vi "HostHoppingScan_v2_IZTracked.vi"() -> ()   [LabVIEW 2024]
uses:
  <vilib>/Analysis/6fits.llb/Curve Fitting Criteria.ctl
  <vilib>/FPGAPlugInAG/USB-7845R OEM/niLvFpga_Open_USB-7845R OEM.vi
  <vilib>/rvi/interface/common/dynamic/niFpgaDynamicAddResources.vi
  <vilib>/Utility/error.llb/Error Cluster From Error Code.vi
  <vilib>/rvi/errors/niLvFpgaAdjustHostInterfaceError.vi
  <vilib>/FPGAPlugInAG/Dynamic/niLvFpga_Close_Dynamic.vi
  <vilib>/rvi/interface/common/niFpgaWaitOnOcc.vi
  <vilib>/rvi/interface/nirviOpenFPGA/nirviOpenFPGA.xnode
  FPGA Bitfiles/hoppingsicmv2_FPGATarget_FPGAScanningPrev_WLYS+VaKxTE.lvbitx
  <vilib>/rvi/interface/nirviReadWriteControl/nirviReadWriteControl.xnode
  <vilib>/rvi/interface/nirviCloseFPGA/nirviCloseFPGA.xnode
  FPGA Bitfiles/hoppingsicmv2_FPGATarget_FPGAHoppingScan_NADRfbve61k.lvbitx
  <vilib>/rvi/interface/nirviMethod/nirviMethod.xnode
  NiFpgaLv.dll
  <vilib>/rvi/interface/Simulation/niFpgaSimulationCallBeginRW.vi
  <vilib>/rvi/errors/niLvFpgaMergeErrorWithErrorCode.vi
  <vilib>/FPGAPlugInAG/Dynamic/niLvFpga_ReadFifo_Dynamic.vi
  <vilib>/FPGAPlugInAG/Dynamic/niLvFpga_WriteFifo_Dynamic.vi
  <vilib>/Analysis/NI_AALPro.lvlib
  <vilib>/FPGAPlugInAG/Dynamic/niLvFpga_ConfigureFifo_Dynamic.vi
panel:
  in  "SubstrateReference?":bool
  out "Signal Size":i32
  in  "Halting Threshold %":dbl format="%#_13g"
  in  "ScanPreview?":bool
  out "Done?":bool
  out "HTT_Buffer_Write":u32
  out "Scanned Points":i32
  in  "stop":bool
  in  "Notes":string
  in  "Pressure kPa":dbl format="%#_13g"
  in  "GraphTab":T1(tab)
  out "Topography":dbl[][](graph)
  out "IZCurve":cluster{dbl[], dbl[]}(graph)
  out "Pressure Slope Map":dbl[][](graph)
  out "FPGA_Host_Buf_Depth":u32
  in  "NF_AppRate um/s":dbl format="%#_13g"
  in  "FF_AppRate um/s":dbl format="%#_13g"
  in  "RetRate um/s":dbl format="%#_13g"
  in  "Retract um":dbl format="%#_13g"
  in  "XOffset um":dbl format="%#_13g"
  in  "YOffset um":dbl format="%#_13g"
  in  "YStepSize um":dbl format="%#_13g"
  in  "XStepSize um":dbl format="%#_13g"
  in  "Recording Threshold %":dbl format="%#_13g"
  in  "YNum":i32
  in  "XNum":i32
  in  "FrameNum":u32
  # "Put this down! ^^^"
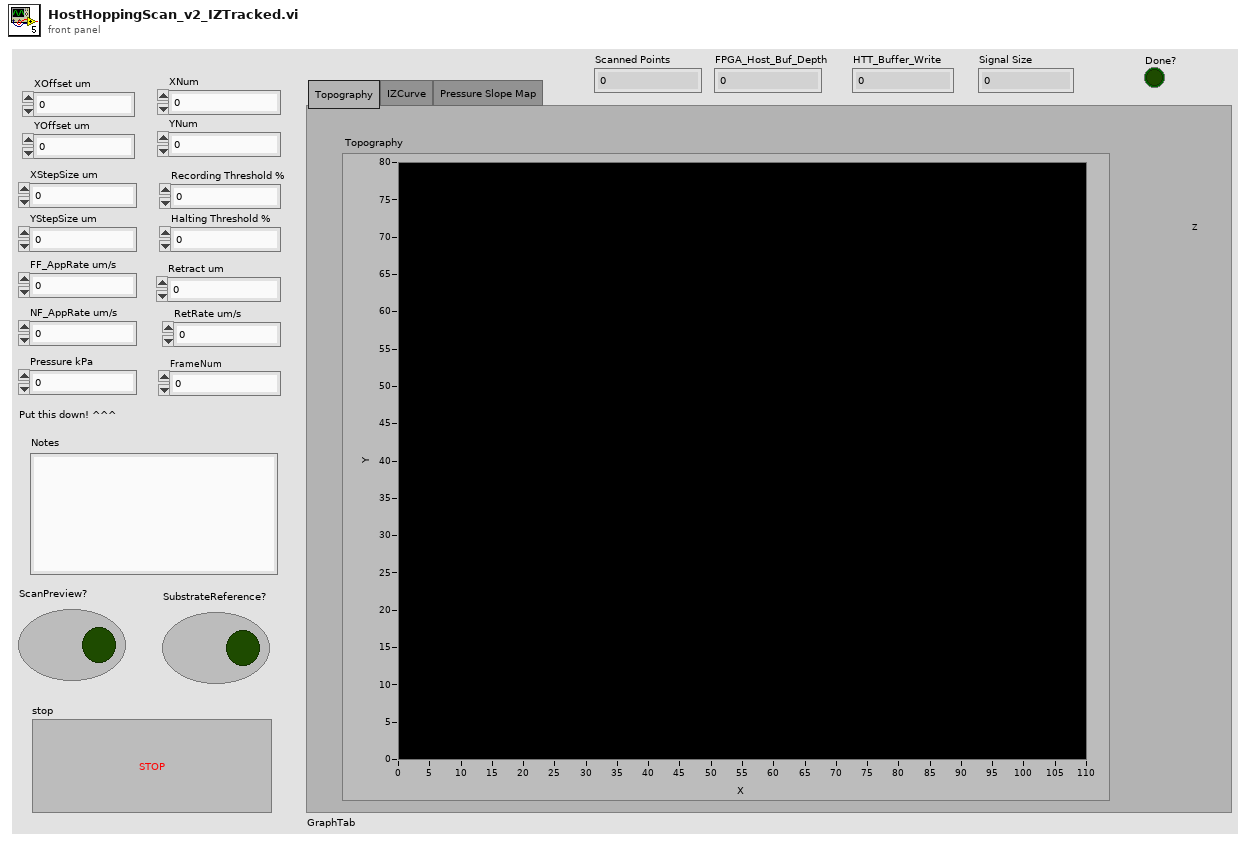
[diagram p1: front panel]
types:
  T1 = enum32{"Topography", "IZCurve", "Pressure Slope Map"}
  T2 = typedef "NI_AALPro.lvlib/Curve Fitting Criteria.ctl" = u16
diagram:
  n1 = flat-sequence {
    tunnel: [w4] -> w2
    tunnel: w2 -> [w14]
    tunnel: [w10] -> w1
    tunnel: w1 -> [w841]
    frame #0 {
      n2 = Obtain Queue(max queue size (-1, unlimited)=64, name (unnamed)="stop_sign", element data type=FALSE) -> (queue out=w4:refnum<queue>)  [unwired: 2 in, 2 out]
    }
    frame #1 {
      n3 = flat-sequence {
        tunnel: [w33] -> w15
        tunnel: w14 -> [w33]
        tunnel: w15 -> [w40]
        tunnel: [w40] -> w8
        tunnel: w8 -> [w104]
        tunnel: [w105] -> w7
        tunnel: [w114] -> w24
        tunnel: w7 -> [w113]
        tunnel: [w113] -> w13
        tunnel: w24 -> [w142]
        tunnel: [w124] -> w23
        tunnel: [w123] -> w22
        tunnel: [w121] -> w21
        tunnel: [w120] -> w20
        tunnel: w13 -> [w118]
        tunnel: [w118] -> w12
        tunnel: w23 -> [w155]
        tunnel: w22 -> [w154]
        tunnel: w21 -> [w153]
        tunnel: [w151] -> w19
        tunnel: [w150] -> w18
        tunnel: [w149] -> w17
        tunnel: [w148] -> w16
        tunnel: w20 -> [w152]
        tunnel: w12 -> [w147]
        tunnel: [w146] -> w11
        tunnel: w19 -> [w821]
        tunnel: w18 -> [w833]
        tunnel: w17 -> [w832]
        tunnel: w16 -> [w831]
        tunnel: w11 -> [w819]
        tunnel: [w819] -> w9
        tunnel: [w840] -> w10
        tunnel: w9 -> [w840]
        frame #0 {
          n4 = Wait (ms)(milliseconds to wait=u32 100) -> ()  [unwired: 1 out]
          "Done?" <- FALSE ("Done?")
        }
        frame #1 {
          n5 = local read "ScanPreview?"() -> (w35:bool)
          n6 = Get Queue Status(queue=w40) -> (queue out=w36:refnum<queue>, # elements in queue=w39:i32)  [unwired: 2 in, 6 out]
          n7 = Less Or Equal To 0?(x=w39) -> (x <= 0?=w38:bool)
          n8 = And(x=w35, y=w38) -> (x .and. y?=w37:bool)
          n9 = case shown="True" w37 {
            tunnel: w36 -> [_ w48]
            frame False {
            }
            frame True {
              n10 = flat-sequence {
                tunnel: w48 -> [w57]
                tunnel: [w56] -> w47
                tunnel: [w55] -> w46
                tunnel: [w57] -> w45
                tunnel: w47 -> [w83]
                tunnel: w46 -> [w82]
                tunnel: w45 -> [w84]
                tunnel: [w81] -> w44
                tunnel: [w80] -> w43
                tunnel: w44 -> [w97]
                tunnel: w43 -> [w96]
                tunnel: [w97] -> w42
                tunnel: [w96] -> w41
                tunnel: w42 -> [w100]
                tunnel: w41 -> [w99]
                frame #0 {
                  n11 = local read "YStepSize um"() -> (w61:dbl)
                  n12 = local read "XStepSize um"() -> (w69:dbl)
                  n13 = local read "YNum"() -> (w62:i32)
                  n14 = local read "XNum"() -> (w68:i32)
                  n15 = local read "XOffset um"() -> (w65:dbl)
                  n16 = local read "YOffset um"() -> (w60:dbl)
                  n17 = xnode "Open FPGA VI Reference"("resource name"=tag "RIO0") -> ("FPGA VI Reference Out"=w78:refnum<k20>, "error out"=w77:errorcluster)  [unwired: 1 in]
                  n18 = Decrement(x=w62) -> (x-1=w63:i32)
                  n19 = Decrement(x=w68) -> (x-1=w67:i32)
                  n20 = Multiply(x=w63, y=w61) -> (x*y=w64:dbl)
                  n21 = Multiply(x=w67, y=w69) -> (x*y=w66:dbl)
                  n22 = Add(x=w60, y=w64) -> (x+y=w50:dbl)
                  n23 = Add(x=w65, y=w66) -> (x+y=w53:dbl)
                  n24 = Divide(x=w50, y=10.0) -> (x/y=w49:dbl)
                  n25 = Divide(x=w53, y=10.0) -> (x/y=w52:dbl)
                  n26 = Divide(x=w60, y=10.0) -> (x/y=w72:dbl)
                  n27 = Divide(x=w65, y=10.0) -> (x/y=w74:dbl)
                  n28 = To Fixed-Point(number=w72) -> (fixed-point=w71:fxp<+/-,48,16>)  [unwired: 1 in]
                  n29 = To Fixed-Point(number=w49) -> (fixed-point=w58:fxp<+/-,48,16>)  [unwired: 1 in]
                  n30 = To Fixed-Point(number=w74) -> (fixed-point=w73:fxp<+/-,48,16>)  [unwired: 1 in]
                  n31 = To Fixed-Point(number=w52) -> (fixed-point=w59:fxp<+/-,48,16>)  [unwired: 1 in]
                  n32 = xnode "Read/Write Control"("FPGA VI Reference In"=w78, "error in"=w77, "X_start"=w73, "X_end"=w59, "Y_start"=w71, "Y_end"=w58, "rate us"=75) -> ("FPGA VI Reference Out"=w56:refnum<k20>, "error out"=w55:errorcluster)
                }
                frame #1 {
                  n33 = while {
                    tunnel: w84 -> [w95]
                    tunnel: w83 -> [w93]
                    tunnel: w82 -> [w92]
                    tunnel: [w91] -> w81
                    tunnel: [w90] -> w80
                    stop <- w85 stop-if-true
                    n34 = local read "ScanPreview?"() -> (w89:bool)
                    n35 = Get Queue Status(queue=w95) -> (# elements in queue=w94:i32)  [unwired: 2 in, 7 out]
                    n36 = Greater Than 0?(x=w94) -> (x > 0?=w88:bool)
                    n37 = Compound Arithmetic op=OR(invert w89, w88) -> (w87:bool)
                    n38 = xnode "Read/Write Control"("FPGA VI Reference In"=w93, "error in"=w92, "stop"=w87) -> ("FPGA VI Reference Out"=w91:refnum<k20>, "error out"=w90:errorcluster, "TargetDone?"=w85:bool)
                    n39 = Wait (ms)(milliseconds to wait=u32 10) -> ()  [unwired: 1 out]
                  }
                }
                frame #2 {
                  n40 = Wait (ms)(milliseconds to wait=u32 100) -> ()  [unwired: 1 out]
                }
                frame #3 {
                  n41 = xnode "Close FPGA VI Reference"("FPGA VI Reference In"=w100, "error in"=w99) -> ()  [unwired: 1 out]
                }
              }
            }
          }
        }
        frame #2 {
          n42 = Get Queue Status(queue=w104) -> (queue out=w103:refnum<queue>, # elements in queue=w102:i32)  [unwired: 2 in, 6 out]
          n43 = Greater Than 0?(x=w102) -> (x > 0?=w101:bool)
          n44 = case shown="True" w101 {
            tunnel: w103 -> [w107 w110]
            tunnel: [w107 w108] -> w105
            frame False {
            }
            frame True {
              n45 = flat-sequence {
                tunnel: w110 -> [w111]
                tunnel: [w111] -> w109
                tunnel: w109 -> [w112]
                tunnel: [w112] -> w108
                frame #0 {
                  n46 = Release Queue(queue=w111) -> ()  [unwired: 2 in, 3 out]
                }
                frame #1 {
                  n47 = Stop() -> ()  [unwired: 1 in]
                }
              }
            }
          }
          n48 = Wait (ms)(milliseconds to wait=u32 200) -> ()  [unwired: 1 out]
        }
        frame #3 {
          n49 = call "File Dialog"("prompt"="Choose a path to save scanning image data files") -> ("selected path"=w114:path, "cancelled"=w116:bool, "error out"=w115:errorcluster)  [unwired: 11 in, 1 out]
          n50 = Stop(stop? (T)=w116) -> ()
          n51 = call <vilib>:"Clear Errors.vi"("error in (no error)"=w115) -> ()  [unwired: 5 in, 2 out]
        }
        frame #4 {
          w127 = refnum<k38> refnum  # db_object
          # "use python to save data this time"
          n52 = Path To String(path=w142) -> (string=w141:string)
          n53 = Concatenate Strings(w141, "_data.db" ("string")) -> (w140:string)
          n54 = String To Path(string=w140) -> (path=w138:path)
          n55 = call <vilib>:"Check if File or Folder Exists.vi"("path"=w138) -> ("file or folder exists?"=w139:bool)  [unwired: 8 in, 2 out]
          n56 = Current VI's Path() -> (path=w132:path)
          n57 = case shown="True" w139 {
            tunnel: w138 -> [w143 w145]
            tunnel: [w143 w144] -> w137
            frame False {
            }
            frame True {
              n58 = Delete(path (use dialog)=w145) -> (deleted path=w144:path)  [unwired: 4 in, 2 out]
            }
          }
          n59 = Strip Path(path=w132) -> (stripped path=w131:path)  [unwired: 1 out]
          n60 = Path To String(path=w137) -> (string=w128:string)
          n61 = Build Path(base path=w131, name or relative path=path "py/data_db_arrangement.py") -> (appended path=w120:path)
          n62 = Open Python Session(python version="3.9" ("Python version")) -> (session out=w134:refnum<k35>, error out=w133:errorcluster)  [unwired: 2 in]
          n63 = node(w134, w120, "db_init" ("Python version"), w133, w127, w128) -> (w126:refnum<k35>, w125:errorcluster, w122:refnum<k38>)  [unwired: 1 in, 2 out]
          n64 = node(w126, w120, "db_start_global_timer" ("function name"), w125, w122) -> (w124:refnum<k35>, w123:errorcluster, w121:refnum<k38>)  [unwired: 2 in, 2 out]
        }
        frame #5 {
          n65 = local read "FrameNum"() -> (w156:u32)
          n66 = for {
            N: w156 -> [_]
            tunnel: w155 -> [w183]
            tunnel: w154 -> [w182]
            tunnel: w153 -> [w181]
            tunnel: w152 -> [w180]
            tunnel: [w169] -> w151
            tunnel: [w168] -> w150
            tunnel: [w167] -> w149
            tunnel: [w166] -> w148
            tunnel: w147 -> [w162]
            tunnel: [w159] -> w146
            i -> [w179]
            stop <- w163 stop-if-true
            n67 = flat-sequence {
              tunnel: w179 -> [w197]
              tunnel: w180 -> [w190]
              tunnel: w181 -> [w192]
              tunnel: w182 -> [w193]
              tunnel: w183 -> [w194]
              tunnel: [w191] -> w178
              tunnel: [w189] -> w177
              tunnel: [w188] -> w176
              tunnel: [w190] -> w175
              tunnel: [w197] -> w174
              tunnel: w162 -> [w186]
              tunnel: [w186] -> w161
              tunnel: [w237] -> w184
              tunnel: w178 -> [w232]
              tunnel: w177 -> [w231]
              tunnel: w176 -> [w230]
              tunnel: w175 -> [w229]
              tunnel: w174 -> [w228]
              tunnel: [w223] -> w173
              tunnel: [w222] -> w172
              tunnel: [w221] -> w171
              tunnel: [w220] -> w170
              tunnel: [w219] -> w165
              tunnel: [w218] -> w164
              tunnel: w161 -> [w208]
              tunnel: [w207] -> w160
              tunnel: [w203] -> w158
              tunnel: [w202] -> w157
              tunnel: w184 -> [w810]
              tunnel: w173 -> [w805]
              tunnel: w172 -> [w807]
              tunnel: w171 -> [w806]
              tunnel: w170 -> [w802]
              tunnel: [w805] -> w169
              tunnel: [w804] -> w168
              tunnel: [w803] -> w167
              tunnel: [w801] -> w166
              tunnel: w165 -> [w808]
              tunnel: w164 -> [w809]
              tunnel: [w809] -> w163
              tunnel: w160 -> [w799]
              tunnel: [w799] -> w159
              tunnel: w158 -> [w797]
              tunnel: w157 -> [w798]
              frame #0 {
                w185 = FALSE ("Y Scale.Loose Fit")
                n68 = local read "XNum"() -> (w196:i32)
                n69 = local read "YNum"() -> (w195:i32)
                n70 = property on="Pressure Slope Map" class="IntGraph (strict)"("XScale.Maximum"=w196, "YScale.Maximum"=w195, "YScale.LooseFit"=w185, "XScale.LooseFit"=w185, "ZScale.LooseFit"=w185) -> ()  [unwired: 2 in, 2 out]
                n71 = property on="Topography" class="IntGraph (strict)"("XScale.Maximum"=w196, "YScale.Maximum"=w195, "YScale.LooseFit"=w185, "XScale.LooseFit"=w185, "ZScale.LooseFit"=w185) -> ()  [unwired: 2 in, 2 out]
                n72 = node(w194, w190, "db_start_frame_timer" ("function name"), w193, w192) -> (w191:refnum<k35>, w189:errorcluster, w188:refnum<k38>)  [unwired: 2 in, 2 out]
              }
              frame #1 {
                w200 = 100000.0
                w201 = -100000.0
                # "TTH param structure:\n0, 1: X, Y piezo voltage\n2, 3: X, Y piezo idx\n4: Z piezo voltage\n5: baseline current\n(6-8105): Z voltage\n(8106-16205): current"
                # "HTT param structure:\n0, 1: X, Y piezo voltage\n2, 3: X, Y piezo idx\n4: distance (piezo voltage) to the last point\n5: retract height, \nall negative cases won't trigger approach of z piezo\nif -20, keep z and move xy\nif -30, full retract for z and move xy"
                n73 = Obtain Queue(name (unnamed)="data_array", element data type=dbl[] []) -> (queue out=w233:refnum<queue>)  [unwired: 3 in, 2 out]
                n74 = New Data Value Reference(data value=FALSE) -> (data value reference=w234:refnum<data-value>)  [unwired: 1 in, 1 out]
                n75 = local read "XNum"() -> (w226:i32)
                n76 = local read "YNum"() -> (w225:i32)
                n77 = Initialize Array(0.0, w226, w225) -> (w224:dbl[][])
                n78 = flat-sequence {
                  tunnel: w234 -> [w560]
                  tunnel: w233 -> [w561]
                  tunnel: [w561] -> w258
                  tunnel: [w560] -> w256
                  tunnel: [w559] -> w254
                  tunnel: [w551] -> w251
                  tunnel: [w545] -> w245
                  tunnel: [w542] -> w244
                  tunnel: [w536] -> w243
                  tunnel: [w533] -> w242
                  tunnel: [w532] -> w199
                  tunnel: [w522] -> w198
                  tunnel: [w583] -> w260
                  tunnel: [w582] -> w259
                  tunnel: w258 -> [w581]
                  tunnel: [w581] -> w257
                  tunnel: w256 -> [w574]
                  tunnel: [w574] -> w255
                  tunnel: w254 -> [w564]
                  tunnel: [w576] -> w253
                  tunnel: [w575] -> w252
                  tunnel: w251 -> [w573]
                  tunnel: [w573] -> w250
                  tunnel: [w574] -> w249
                  tunnel: [w572] -> w248
                  tunnel: [0] -> w247
                  tunnel: [w570] -> w246
                  tunnel: w245 -> [w569]
                  tunnel: w244 -> [w568]
                  tunnel: w243 -> [w567]
                  tunnel: w242 -> [w565]
                  tunnel: [0] -> w236
                  tunnel: [w565] -> w235
                  tunnel: w199 -> [w563]
                  tunnel: w198 -> [w562]
                  tunnel: w260 -> [w609]
                  tunnel: w259 -> [w608]
                  tunnel: w257 -> [w607]
                  tunnel: w255 -> [w606]
                  tunnel: w253 -> [w605]
                  tunnel: w252 -> [w604]
                  tunnel: w250 -> [w603]
                  tunnel: w249 -> [w602]
                  tunnel: w248 -> [w601]
                  tunnel: w247 -> [w600]
                  tunnel: w246 -> [w599]
                  tunnel: [w598] -> w241
                  tunnel: [w597] -> w240
                  tunnel: [w596] -> w239
                  tunnel: [w595] -> w238
                  tunnel: w236 -> [w594]
                  tunnel: w235 -> [w593]
                  tunnel: [w592] -> w217
                  tunnel: [w591] -> w206
                  tunnel: [w775] -> w216
                  tunnel: [w774] -> w214
                  tunnel: [w773] -> w212
                  tunnel: [w771] -> w210
                  tunnel: w217 -> [w770]
                  tunnel: w238 -> [w772]
                  tunnel: w239 -> [w773]
                  tunnel: w240 -> [w774]
                  tunnel: w241 -> [w775]
                  tunnel: w206 -> [w769]
                  tunnel: [w769] -> w204
                  tunnel: w216 -> [w789]
                  tunnel: [w789] -> w215
                  tunnel: w214 -> [w788]
                  tunnel: [w788] -> w213
                  tunnel: w212 -> [w787]
                  tunnel: [w787] -> w211
                  tunnel: w210 -> [w786]
                  tunnel: [w786] -> w209
                  tunnel: [w784] -> w205
                  tunnel: w204 -> [w784]
                  tunnel: w215 -> [w794]
                  tunnel: w213 -> [w793]
                  tunnel: w211 -> [w795]
                  tunnel: w209 -> [w792]
                  tunnel: [w792] -> w237
                  tunnel: [w791] -> w219
                  tunnel: w205 -> [w790]
                  tunnel: [w790] -> w203
                  frame #0 {
                    n79 = local read "NF_AppRate um/s"() -> (w543:dbl)
                    n80 = local read "FF_AppRate um/s"() -> (w548:dbl)
                    n81 = local read "Recording Threshold %"() -> (w531:dbl)
                    n82 = local read "SubstrateReference?"() -> (w525:bool)
                    n83 = local read "Halting Threshold %"() -> (w527:dbl)
                    n84 = local read "RetRate um/s"() -> (w538:dbl)
                    n85 = local read "XNum"() -> (w535:i32)
                    n86 = local read "YNum"() -> (w534:i32)
                    n87 = Divide(x=25.0, y=0.032768) -> (x/y=w537:dbl)
                    n88 = local read "XStepSize um"() -> (w556:dbl)
                    n89 = local read "YStepSize um"() -> (w555:dbl)
                    n90 = local read "YOffset um"() -> (w554:dbl)
                    n91 = local read "Retract um"() -> (w552:dbl)
                    n92 = local read "XOffset um"() -> (w553:dbl)
                    n93 = local read "XNum"() -> (w558:i32)
                    n94 = local read "YNum"() -> (w557:i32)
                    n95 = Multiply(x=w535, y=w534) -> (x*y=w533:i32)
                    n96 = Divide(x=w531, y=100.0) -> (x/y=w530:dbl)
                    n97 = Divide(x=w527, y=100.0) -> (x/y=w526:dbl)
                    n98 = Divide(x=w537, y=w543) -> (x/y=w539:dbl)
                    n99 = Divide(x=w537, y=w538) -> (x/y=w541:dbl)
                    n100 = Divide(x=w537, y=w548) -> (x/y=w547:dbl)
                    n101 = Round To Nearest(number=w539) -> (nearest integer value=w544:dbl)
                    n102 = Round To Nearest(number=w541) -> (nearest integer value=w540:dbl)
                    n103 = Round To Nearest(number=w547) -> (nearest integer value=w546:dbl)
                    n104 = To Fixed-Point(number=w530) -> (fixed-point=w559:fxp<+/-,48,16>)  [unwired: 1 in]
                    n105 = To Fixed-Point(number=w526) -> (fixed-point=w532:fxp<+/-,48,16>)  [unwired: 1 in]
                    n106 = call "xy_raster_scan.vi"("Retract um"=w552, "YOffset um"=w554, "XOffset um"=w553, "YStepSize um"=w555, "XStepSize um"=w556, "YNum"=w557, "XNum"=w558) -> ("Converted_HTT_Params"=w551:fxp<+/-,48,16>[])  [unwired: 4 in]
                    n107 = Select(t=2, s=w525, f=1) -> (s? t:f=w522:i32)
                    n108 = To Long Integer(number=w544) -> (32bit integer=w542:i32)
                    n109 = To Long Integer(number=w540) -> (32bit integer=w536:i32)
                    n110 = To Long Integer(number=w546) -> (32bit integer=w545:i32)
                  }
                  frame #1 {
                    n111 = xnode "Open FPGA VI Reference"("resource name"=tag "RIO0") -> ("FPGA VI Reference Out"=w580:refnum<k20>, "error out"=w579:errorcluster)  [unwired: 1 in]
                    n112 = xnode "Read/Write Control"("FPGA VI Reference In"=w580, "error in"=w579, "Recording Threshold"=w564, "Halting Threshold"=w563, "AppRate_FF us"=w569, "AppRate_NF us"=w568, "RetRate us"=w567, "TotalPoints"=w565, "DelayPoints"=w562) -> ("FPGA VI Reference Out"=w589:refnum<k20>, "error out"=w588:errorcluster)
                    n113 = xnode "Invoke Method"("FPGA VI Reference In"=w580, "error in"=w579, "Data"=fxp<+/-,48,16>[] [], "Timeout (ms)"=0) -> ("FPGA VI Reference Out"=w576:refnum<k20>, "error out"=w575:errorcluster, "Empty Elements Remaining"=w570:u32)
                    n114 = Scale By Power Of 2(n=u32 18 ("Requested Depth"), x=u32 1 ("Requested Depth")) -> (x*2^n=w585:u32)
                    n115 = xnode "Invoke Method"("FPGA VI Reference In"=w589, "error in"=w588, "Requested Depth"=w585) -> ("FPGA VI Reference Out"=w583:refnum<k20>, "error out"=w582:errorcluster, "Actual Depth"=→"FPGA_Host_Buf_Depth":u32)
                    n116 = Array Size(array=w573) -> (size(s)=w572:i32)
                  }
                  frame #2 {
                    n117 = while {
                      tunnel: w605 -> [w627]
                      tunnel: w604 -> [w626]
                      tunnel: w603 -> [w623]
                      tunnel: w602 -> [w622]
                      tunnel: w601 -> [w621]
                      shift-right: [w614] -> _
                      shift-left: w600 -> [w620]
                      tunnel: w599 -> [w619]
                      stop <- w610 stop-if-true
                      n118 = flat-sequence {
                        tunnel: w627 -> [w651]
                        tunnel: w626 -> [w650]
                        tunnel: [w645] -> w625
                        tunnel: [w644] -> w624
                        tunnel: w623 -> [w633]
                        tunnel: w622 -> [w643]
                        tunnel: w621 -> [w642]
                        tunnel: w620 -> [w637]
                        tunnel: w619 -> [w641]
                        tunnel: [w637] -> w618
                        tunnel: [w634] -> w617
                        tunnel: [w633] -> w616
                        tunnel: [w629] -> w613
                        tunnel: [w628] -> w612
                        tunnel: w625 -> [w660]
                        tunnel: w624 -> [w659]
                        tunnel: w618 -> [w658]
                        tunnel: w617 -> [w657]
                        tunnel: w616 -> [w656]
                        tunnel: [w655] -> w615
                        tunnel: w613 -> [w654]
                        tunnel: w612 -> [w653]
                        tunnel: [w653] -> w611
                        tunnel: w615 -> [w671]
                        tunnel: [w671] -> w614
                        tunnel: w611 -> [w670]
                        tunnel: [w670] -> w610
                        frame #0 {
                          w635 = u32 128 ("y")
                          n119 = in-place {
                            in-place-border: [w652] -> w631
                            n120 = in-place-dvr #1(w643) -> (w652:bool)  [unwired: 1 out]
                            n121 = in-place-dvr #1(w652) -> ()  [unwired: 2 out]
                          }
                          n122 = xnode "Invoke Method"("FPGA VI Reference In"=w651, "error in"=w650, "Data"=fxp<+/-,48,16>[] [], "Timeout (ms)"=0) -> ("FPGA VI Reference Out"=w647:refnum<k20>, "error out"=w646:errorcluster, "Empty Elements Remaining"=w640:u32)
                          n123 = Subtract(x=w642, y=w637) -> (x-y=w636:u32)
                          n124 = Subtract(x=w641, y=w640) -> (x-y=w639:u32)
                          n125 = Less Or Equal?(x=w639, y=w635) -> (x <= y?=w638:bool)
                          n126 = Less Or Equal?(x=w636, y=w635) -> (x <= y?=w630:bool)
                          n127 = Or(x=w638, y=w630) -> (x .or. y?=w629:bool)
                          n128 = xnode "Read/Write Control"("FPGA VI Reference In"=w647, "error in"=w646) -> ("FPGA VI Reference Out"=w645:refnum<k20>, "error out"=w644:errorcluster, "TargetDone?"=w632:bool)
                          n129 = Select(t=w636, s=w630, f=w635) -> (s? t:f=w634:u32)
                          n130 = Compound Arithmetic op=OR(w632, w630, w631) -> (w628:bool)
                        }
                        frame #1 {
                          n131 = case shown="True" w654 {
                            tunnel: w660 -> [_ w669]
                            tunnel: w659 -> [_ w668]
                            tunnel: w658 -> [w661 w664]
                            tunnel: w657 -> [_ w663]
                            tunnel: w656 -> [_ w665]
                            tunnel: [w661 w666] -> w655
                            frame False {
                            }
                            frame True {
                              n132 = Array Subset(array=w665, index=w664, length=w663) -> (w662:fxp<+/-,48,16>[])
                              n133 = Add(x=w663, y=w664) -> (x+y=w666:u32)
                              "HTT_Buffer_Write" <- w666
                              n134 = xnode "Invoke Method"("FPGA VI Reference In"=w669, "error in"=w668, "Data"=w662, "Timeout (ms)"=10000) -> ()  [unwired: 3 out]
                            }
                          }
                        }
                        frame #2 {
                          n135 = Wait (ms)(milliseconds to wait=u32 100) -> ()  [unwired: 1 out]
                        }
                      }
                    }
                    n136 = while {
                      tunnel: w609 -> [w702]
                      tunnel: w608 -> [w701]
                      tunnel: w607 -> [w698]
                      tunnel: w606 -> [w697]
                      tunnel: [w690] -> w598
                      tunnel: [w689] -> w597
                      tunnel: [w687] -> w596
                      tunnel: [w685] -> w595
                      shift-right: [w681] -> _
                      shift-left: w594 -> [w684]
                      tunnel: w593 -> [w677]
                      tunnel: [w674] -> w592
                      tunnel: [w673] -> w591
                      stop <- w678 stop-if-true
                      n137 = flat-sequence {
                        tunnel: w702 -> [w721]
                        tunnel: w701 -> [w720]
                        tunnel: [w715] -> w700
                        tunnel: [w714] -> w699
                        tunnel: w698 -> [w710]
                        tunnel: w697 -> [w708]
                        tunnel: [w710] -> w696
                        tunnel: [w709] -> w695
                        tunnel: [w707] -> w694
                        tunnel: [w706] -> w691
                        tunnel: w684 -> [w705]
                        tunnel: [w705] -> w683
                        tunnel: [w704] -> w680
                        tunnel: w677 -> [w703]
                        tunnel: [w703] -> w676
                        tunnel: w700 -> [w735]
                        tunnel: w699 -> [w734]
                        tunnel: w696 -> [w733]
                        tunnel: w695 -> [w732]
                        tunnel: w694 -> [w731]
                        tunnel: [w730] -> w693
                        tunnel: [w729] -> w692
                        tunnel: w691 -> [w728]
                        tunnel: [w728] -> w688
                        tunnel: [w727] -> w686
                        tunnel: w683 -> [w726]
                        tunnel: [w725] -> w682
                        tunnel: w680 -> [w724]
                        tunnel: [w724] -> w679
                        tunnel: w676 -> [w723]
                        tunnel: [w723] -> w675
                        tunnel: w693 -> [w767]
                        tunnel: w692 -> [w766]
                        tunnel: [w767] -> w690
                        tunnel: [w766] -> w689
                        tunnel: [w765] -> w687
                        tunnel: w688 -> [w765]
                        tunnel: w686 -> [w764]
                        tunnel: [w764] -> w685
                        tunnel: w682 -> [w762]
                        tunnel: [w762] -> w681
                        tunnel: w679 -> [w760]
                        tunnel: [w763] -> w678
                        tunnel: w675 -> [w761]
                        tunnel: [w760] -> w674
                        tunnel: [w759] -> w673
                        frame #0 {
                          w713 = 16384
                          w717 = u32 0 ("Number of Elements")
                          n138 = in-place {
                            in-place-border: [w722] -> w704
                            n139 = in-place-dvr #2(w708) -> (w722:bool)  [unwired: 1 out]
                            n140 = in-place-dvr #2(w722) -> (w706:refnum<data-value>)  [unwired: 1 out]
                          }
                          n141 = xnode "Read/Write Control"("FPGA VI Reference In"=w721, "error in"=w720, "stop"=w704) -> ("FPGA VI Reference Out"=w719:refnum<k20>, "error out"=w718:errorcluster)
                          n142 = xnode "Invoke Method"("FPGA VI Reference In"=w719, "error in"=w718, "Number of Elements"=w717, "Timeout (ms)"=w717) -> ("FPGA VI Reference Out"=w715:refnum<k20>, "error out"=w714:errorcluster, "Elements Remaining"=w716:u32)  [unwired: 1 out]
                          n143 = Quotient & Remainder(x=w716, y=w713) -> (floor(x/y)=w712:u32)  [unwired: 1 out]
                          n144 = Multiply(x=w713, y=w712) -> (x*y=w707:u32)
                          n145 = Greater Than 0?(x=w712) -> (x > 0?=w711:bool)
                          n146 = Compound Arithmetic op=AND(w711, invert w704) -> (w709:bool)
                        }
                        frame #1 {
                          n147 = case shown="True" w732 {
                            tunnel: w735 -> [w739 w755]
                            tunnel: w734 -> [w738 w754]
                            tunnel: w733 -> [w737 w748]
                            tunnel: w731 -> [_ w750]
                            tunnel: [w739 w752] -> w730
                            tunnel: [w738 w751] -> w729
                            tunnel: [w737 w743] -> w727
                            tunnel: w726 -> [w736 w742]
                            tunnel: [w736 w740] -> w725
                            frame False {
                            }
                            frame True {
                              w745 = 16384
                              n148 = xnode "Invoke Method"("FPGA VI Reference In"=w755, "error in"=w754, "Number of Elements"=w750, "Timeout (ms)"=10000) -> ("FPGA VI Reference Out"=w752:refnum<k20>, "error out"=w751:errorcluster, "Data"=w749:fxp<+/-,48,16>[])  [unwired: 1 out]
                              n149 = To Double Precision Float(number=w749) -> (double precision float=w746:dbl[])
                              n150 = Array Size(array=w746) -> (size(s)=w747:i32)
                              n151 = Quotient & Remainder(x=w747, y=w745) -> (floor(x/y)=w741:i32)  [unwired: 1 out]
                              n152 = Add(x=w742, y=w741) -> (x+y=w740:i32)
                              n153 = Reshape Array(w746, w741, w745) -> (w744:dbl[][])
                              n154 = for {
                                N: w741 -> [_]
                                tunnel: w748 -> [w758]
                                tunnel: w744 -> [w757] mode=indexing
                                tunnel: [w756] -> w743
                                n155 = Enqueue Element(queue=w758, element=w757) -> (queue out=w756:refnum<queue>)  [unwired: 2 in, 2 out]
                              }
                            }
                          }
                        }
                        frame #2 {
                          n156 = Greater Or Equal?(x=w762, y=w761) -> (x >= y?=w759:bool)
                          n157 = Wait (ms)(milliseconds to wait=u32 20) -> ()  [unwired: 1 out]
                          n158 = Or(x=w759, y=w760) -> (x .or. y?=w763:bool)
                          "Scanned Points" <- w762
                        }
                      }
                    }
                  }
                  frame #3 {
                    n159 = case shown="False" w770 {
                      tunnel: w772 -> [w777 w783]
                      tunnel: [w776 w783] -> w771
                      frame False {
                        n160 = while {
                          tunnel: w777 -> [w782]
                          tunnel: [w781] -> w776
                          stop <- w779 stop-if-true
                          n161 = Get Queue Status(queue=w782) -> (queue out=w781:refnum<queue>, # elements in queue=w780:i32)  [unwired: 2 in, 6 out]
                          n162 = Less Or Equal To 0?(x=w780) -> (x <= 0?=w779:bool)
                          n163 = Wait (ms)(milliseconds to wait=u32 100) -> ()  [unwired: 1 out]
                        }
                      }
                      frame True {
                      }
                    }
                  }
                  frame #4 {
                    n164 = Wait (ms)(milliseconds to wait=u32 500) -> ()  [unwired: 1 out]
                  }
                  frame #5 {
                    n165 = in-place {
                      n166 = in-place-dvr #3(w795) -> ()  [unwired: 2 out]
                      n167 = in-place-dvr #3(TRUE ("data value")) -> (w791:refnum<data-value>)  [unwired: 1 out]
                    }
                    n168 = xnode "Close FPGA VI Reference"("FPGA VI Reference In"=w794, "error in"=w793) -> ()  [unwired: 1 out]
                  }
                }
                n169 = flat-sequence {
                  tunnel: w234 -> [w284]
                  tunnel: w233 -> [w283]
                  tunnel: w232 -> [w282]
                  tunnel: w231 -> [w281]
                  tunnel: w230 -> [w280]
                  tunnel: w229 -> [w279]
                  tunnel: [w278] -> w223
                  tunnel: [w277] -> w222
                  tunnel: [w276] -> w221
                  tunnel: [w275] -> w220
                  tunnel: w228 -> [w274]
                  tunnel: w224 -> [w273]
                  tunnel: w224 -> [w272]
                  tunnel: w201 -> [w271]
                  tunnel: w200 -> [w270]
                  tunnel: w201 -> [w269]
                  tunnel: w200 -> [w268]
                  tunnel: [w267] -> w218
                  tunnel: w208 -> [w266]
                  tunnel: [w265] -> w207
                  tunnel: [w264] -> w202
                  frame #0 {
                    n170 = while {
                      tunnel: w284 -> [w343]
                      tunnel: w283 -> [w342]
                      tunnel: w282 -> [w341]
                      tunnel: w281 -> [w340]
                      tunnel: w280 -> [w339]
                      tunnel: w279 -> [w335]
                      tunnel: [w329] -> w278
                      tunnel: [w328] -> w277
                      tunnel: [w327] -> w276
                      tunnel: [w326] -> w275
                      tunnel: w274 -> [w322]
                      shift-right: [w312] -> _
                      shift-left: w273 -> [w320]
                      shift-right: [w310] -> _
                      shift-left: w272 -> [w315]
                      shift-right: [w300] -> _
                      shift-left: w271 -> [w309]
                      shift-right: [w298] -> _
                      shift-left: w270 -> [w308]
                      shift-right: [w296] -> _
                      shift-left: w269 -> [w305]
                      shift-right: [w294] -> _
                      shift-left: w268 -> [w304]
                      tunnel: [w291] -> w267
                      tunnel: w266 -> [w290]
                      tunnel: [w287] -> w265
                      tunnel: [w285] -> w264
                      stop <- w317 stop-if-true
                      n171 = flat-sequence {
                        tunnel: w343 -> [w365]
                        tunnel: w342 -> [w360]
                        tunnel: w341 -> [w364]
                        tunnel: w340 -> [w363]
                        tunnel: w339 -> [w362]
                        tunnel: [w364] -> w338
                        tunnel: [w363] -> w337
                        tunnel: [w362] -> w336
                        tunnel: w335 -> [w361]
                        tunnel: [w361] -> w334
                        tunnel: [w359] -> w325
                        tunnel: [w358] -> w324
                        tunnel: [w357] -> w323
                        tunnel: w322 -> [w356]
                        tunnel: [w356] -> w321
                        tunnel: w320 -> [w354]
                        tunnel: [w355] -> w319
                        tunnel: [w354] -> w316
                        tunnel: w315 -> [w353]
                        tunnel: [w353] -> w314
                        tunnel: w309 -> [w352]
                        tunnel: w308 -> [w351]
                        tunnel: [w352] -> w307
                        tunnel: [w351] -> w306
                        tunnel: w305 -> [w350]
                        tunnel: w304 -> [w349]
                        tunnel: [w350] -> w303
                        tunnel: [w349] -> w302
                        tunnel: [w348] -> w293
                        tunnel: w290 -> [w347]
                        tunnel: [w344] -> w289
                        tunnel: w338 -> [w396]
                        tunnel: w337 -> [w395]
                        tunnel: w336 -> [w394]
                        tunnel: w334 -> [w393]
                        tunnel: [w392] -> w333
                        tunnel: [w391] -> w332
                        tunnel: [w390] -> w331
                        tunnel: [w389] -> w330
                        tunnel: w325 -> [w388]
                        tunnel: w324 -> [w387]
                        tunnel: w323 -> [w386]
                        tunnel: w321 -> [w385]
                        tunnel: w319 -> [w384]
                        tunnel: [w384] -> w318
                        tunnel: w316 -> [w383]
                        tunnel: w314 -> [w382]
                        tunnel: [w381] -> w313
                        tunnel: [w380] -> w311
                        tunnel: w307 -> [w379]
                        tunnel: w306 -> [w378]
                        tunnel: w303 -> [w377]
                        tunnel: w302 -> [w376]
                        tunnel: [w375] -> w301
                        tunnel: [w374] -> w299
                        tunnel: [w373] -> w297
                        tunnel: [w372] -> w295
                        tunnel: w293 -> [w371]
                        tunnel: [w371] -> w292
                        tunnel: w289 -> [w370]
                        tunnel: [w370] -> w288
                        tunnel: [w369] -> w286
                        tunnel: w333 -> [w519]
                        tunnel: w332 -> [w518]
                        tunnel: w331 -> [w517]
                        tunnel: w330 -> [w520]
                        tunnel: [w520] -> w329
                        tunnel: [w519] -> w328
                        tunnel: [w518] -> w327
                        tunnel: [w517] -> w326
                        tunnel: [w516] -> w317
                        tunnel: w318 -> [w516]
                        tunnel: w313 -> [w515]
                        tunnel: [w515] -> w312
                        tunnel: w311 -> [w514]
                        tunnel: [w514] -> w310
                        tunnel: w301 -> [w513]
                        tunnel: [w513] -> w300
                        tunnel: w299 -> [w512]
                        tunnel: [w512] -> w298
                        tunnel: w297 -> [w511]
                        tunnel: [w511] -> w296
                        tunnel: w295 -> [w510]
                        tunnel: [w510] -> w294
                        tunnel: w292 -> [w509]
                        tunnel: [w509] -> w291
                        tunnel: w288 -> [w508]
                        tunnel: [w508] -> w287
                        tunnel: w286 -> [w507]
                        tunnel: [w507] -> w285
                        frame #0 {
                          # "topography max min"
                          # "pressure slope map"
                          # "topography"
                          n172 = Get Queue Status(queue=w347) -> (queue out=w344:refnum<queue>, # elements in queue=w346:i32)  [unwired: 2 in, 6 out]
                          n173 = Greater Than 0?(x=w346) -> (x > 0?=w345:bool)
                          n174 = Get Queue Status(queue=w360) -> (queue out=w358:refnum<queue>, # elements in queue=w357:i32)  [unwired: 2 in, 6 out]
                          n175 = in-place {
                            in-place-border: w345 -> [w366]
                            in-place-border: [w367] -> w355
                            in-place-border: [w366] -> w348
                            n176 = in-place-dvr #4(w365) -> (w368:bool)  [unwired: 1 out]
                            n177 = Or(x=w368, y=w366) -> (x .or. y?=w367:bool)
                            n178 = in-place-dvr #4(w367) -> ()  [unwired: 2 out]
                          }
                          n179 = Greater Than 0?(x=w357) -> (x > 0?=w359:bool)
                        }
                        frame #1 {
                          n180 = case shown="True" w388 {
                            tunnel: w396 -> [w406 w434]
                            tunnel: w395 -> [w405 w433]
                            tunnel: w394 -> [w404 w432]
                            tunnel: w393 -> [w407 w428]
                            tunnel: [w406 w431] -> w392
                            tunnel: [w405 w430] -> w391
                            tunnel: [w404 w429] -> w390
                            tunnel: [w407 w427] -> w389
                            tunnel: w387 -> [_ w425]
                            tunnel: w386 -> [_ w426]
                            tunnel: w385 -> [w397 w424]
                            tunnel: w383 -> [w403 w423]
                            tunnel: w382 -> [w402 w422]
                            tunnel: [w403 w421] -> w381
                            tunnel: [w402 w420] -> w380
                            tunnel: w379 -> [w401 w416]
                            tunnel: w378 -> [w400 w415]
                            tunnel: w377 -> [w399 w414]
                            tunnel: w376 -> [w398 w413]
                            tunnel: [w401 w412] -> w375
                            tunnel: [w400 w411] -> w374
                            tunnel: [w399 w410] -> w373
                            tunnel: [w398 w409] -> w372
                            tunnel: [w397 w408] -> w369
                            frame False {
                            }
                            frame True {
                              n181 = for {
                                N: w426 -> [_]
                                tunnel: w428 -> [w492]
                                tunnel: [w492] -> w427
                                tunnel: w434 -> [w499]
                                tunnel: [w495] -> w431
                                tunnel: w433 -> [w497]
                                tunnel: [w494] -> w430
                                tunnel: w432 -> [w496]
                                tunnel: [w493] -> w429
                                tunnel: w425 -> [w491]
                                tunnel: w424 -> [w460]
                                shift-right: [w453] -> w421
                                shift-left: w423 -> [w454]
                                shift-right: [w451] -> w420
                                shift-left: w422 -> [w452]
                                tunnel: [w450] -> w419
                                tunnel: [w436] -> w418
                                shift-right: [w448] -> w412
                                shift-left: w416 -> [w449]
                                shift-right: [w445] -> w411
                                shift-left: w415 -> [w447]
                                shift-right: [w441] -> w410
                                shift-left: w414 -> [w444]
                                shift-right: [w440] -> w409
                                shift-left: w413 -> [w443]
                                tunnel: [w439] -> w408
                                w456 = T2 1 items=["Least Square", "Least Absolute Residual", "Bisquare"] ("method")
                                n182 = Dequeue Element(queue=w491) -> (element=w482:dbl[])  [unwired: 2 in, 3 out]
                                n183 = Array Subset(array=w482, index=6, length=8100 ("index")) -> (w475:dbl[])
                                n184 = Array Subset(array=w482, index=8106, length=8100 ("index")) -> (w476:dbl[])
                                n185 = Index Array(array=w482, index #1=0 ("index"), index #2=1 ("index"), index #3=2 ("index"), index #4=3 ("index"), index #5=4 ("index"), index #6=5 ("index")) -> (element #1=w473:dbl, element #2=w471:dbl, element #3=w470:dbl, element #4=w468:dbl, element #5=w466:dbl, element #6=w457:dbl)
                                n186 = Search 1D Array(1D array=w475, element=-100.0) -> (index of element=w474:i32)  [unwired: 1 in]
                                n187 = Equal?(x=w474, y=-1) -> (x = y?=w477:bool)
                                n188 = To Long Integer(number=w470) -> (32bit integer=w438:i32)
                                n189 = To Long Integer(number=w468) -> (32bit integer=w437:i32)
                                n190 = case shown="False" w477 {
                                tunnel: w476 -> [w503 w505]
                                tunnel: w475 -> [w504 w506]
                                tunnel: w474 -> [w500 _]
                                tunnel: [w502 w506] -> w461
                                tunnel: [w501 w505] -> w436
                                frame False {
                                n191 = Split 1D Array(array=w504, index=w500) -> (first subarray=w502:dbl[])  [unwired: 1 out]
                                n192 = Split 1D Array(array=w503, index=w500) -> (first subarray=w501:dbl[])  [unwired: 1 out]
                                }
                                frame True {
                                }
                                }
                                n193 = Multiply(x=w473, y=10.0) -> (x*y=w459:dbl)
                                n194 = Multiply(x=w471, y=10.0) -> (x*y=w458:dbl)
                                n195 = Multiply(x=w466, y=2.5) -> (x*y=w465:dbl)
                                n196 = Subtract(x=25.0, y=w465) -> (x-y=w446:dbl)
                                n197 = Multiply(x=w461, y=2.5) -> (x*y=w455:dbl[])
                                n198 = Array Size(array=w436) -> (size(s)=→"Signal Size":i32)
                                n199 = Subtract(x=25.0, y=w455) -> (x-y=w450:dbl[])
                                n200 = call <vilib>:"Linear Fit.vi"("Y"=w436, "X"=w450, "method"=w456) -> ("slope"=w442:dbl)  [unwired: 8 in, 4 out]
                                n201 = node(w499, w492, "db_insert_data" ("function name"), w497, w496, w460, w459, w458, w438, w437, w446, w457, w450, w436) -> (w495:refnum<k35>, w494:errorcluster, w493:refnum<k38>, w439:i32)  [unwired: 10 in, 2 out]
                                n202 = Max & Min(x=w446, y=w449) -> (max(x,y)=w448:dbl)  [unwired: 1 out]
                                n203 = Max & Min(x=w447, y=w446) -> (min(x,y)=w445:dbl)  [unwired: 1 out]
                                n204 = Max & Min(x=w442, y=w444) -> (max(x,y)=w441:dbl)  [unwired: 1 out]
                                n205 = Max & Min(x=w443, y=w442) -> (min(x,y)=w440:dbl)  [unwired: 1 out]
                                n206 = Replace Array Subset(array=w452, new element=w442, index (row)=w438, index (col)=w437) -> (w451:dbl[][])
                                n207 = Replace Array Subset(array=w454, new element=w446, index (row)=w438, index (col)=w437) -> (w453:dbl[][])
                              }
                              n208 = Bundle(w419, w418) -> (→"IZCurve":cluster{dbl[], dbl[]})  [unwired: 1 in]
                              n209 = local write "Pressure Slope Map"(w420) -> ()
                              n210 = local write "Topography"(w421) -> ()
                            }
                          }
                        }
                        frame #2 {
                          n211 = Wait (ms)(milliseconds to wait=u32 50) -> ()  [unwired: 1 out]
                        }
                      }
                    }
                  }
                }
              }
              frame #2 {
                n212 = Delete Data Value Reference(data value reference=w808) -> ()  [unwired: 1 in, 2 out]
                n213 = Release Queue(queue=w810) -> ()  [unwired: 2 in, 3 out]
                n214 = node(w807, w805, "db_end_frame_timer" ("function name"), w806, w802, w798, w797) -> (w804:refnum<k35>, w803:errorcluster, w801:refnum<k38>)  [unwired: 4 in, 2 out]
              }
            }
          }
        }
        frame #6 {
          n215 = local read "Recording Threshold %"() -> (w818:dbl)
          n216 = local read "Halting Threshold %"() -> (w817:dbl)
          n217 = local read "NF_AppRate um/s"() -> (w814:dbl)
          n218 = local read "FF_AppRate um/s"() -> (w815:dbl)
          n219 = node(w833, w821, "db_end_global_timer" ("function name"), w832, w831) -> (w830:refnum<k35>, w829:errorcluster, w828:refnum<k38>)  [unwired: 2 in, 2 out]
          n220 = local read "Pressure kPa"() -> (w812:dbl)
          n221 = local read "XStepSize um"() -> (w825:dbl)
          n222 = local read "YStepSize um"() -> (w824:dbl)
          n223 = local read "FrameNum"() -> (w813:u32)
          n224 = local read "XOffset um"() -> (w823:dbl)
          n225 = local read "Retract um"() -> (w816:dbl)
          n226 = local read "YOffset um"() -> (w822:dbl)
          n227 = local read "Notes"() -> (w811:string)
          n228 = local read "XNum"() -> (w827:i32)
          n229 = local read "YNum"() -> (w826:i32)
          n230 = node(w830, w821, "db_insert_info" ("function name"), w829, w828, 0, w827, w826, w825, w824, w823, w822, w818, w817, w816, w815, w814, w813, w812, w811) -> (w837:refnum<k35>, w836:errorcluster, w835:refnum<k38>)  [unwired: 17 in, 2 out]
          n231 = Close Python Session(session in=w837, error in=w836) -> ()  [unwired: 1 out]
          n232 = Close Reference(reference=w835) -> ()  [unwired: 1 in, 1 out]
        }
        frame #7 {
          n233 = local write "Done?"(TRUE ("Done?")) -> ()
        }
      }
      n234 = while {
        tunnel: w14 -> [w26]
        stop <- w28 stop-if-true
        n235 = local read "Done?"() -> (w29:bool)
        n236 = Or(x="stop", y=w29) -> (x .or. y?=w28:bool)
        n237 = case shown="True" "stop" {
          tunnel: w26 -> [_ w31]
          tunnel: "stop" -> [_ w30]
          frame False {
          }
          frame True {
            n238 = Lossy Enqueue Element(queue=w31, element=w30) -> ()  [unwired: 1 in, 4 out]
          }
        }
        n239 = Wait (ms)(milliseconds to wait=u32 20) -> ()  [unwired: 1 out]
      }
    }
    frame #2 {
      n240 = Release Queue(queue=w841) -> ()  [unwired: 2 in, 3 out]
    }
  }
